vi "GUI RMM List.vi"(7 "FOFB-Controller IP Address in":string, 8 "error in (no error)":errorcluster, 9 "directory path":string, 10 "username":string, 11 "password":string) -> (0 "error out":errorcluster, 3 "RMM List":string[](array[string]))   [LabVIEW 2011, in "User Interface VIs.lvlib"]
uses:
  User Interface VIs.lvlib
  <vilib>/addons/internet/NI_InternetTK_FTP_VIs.lvlib
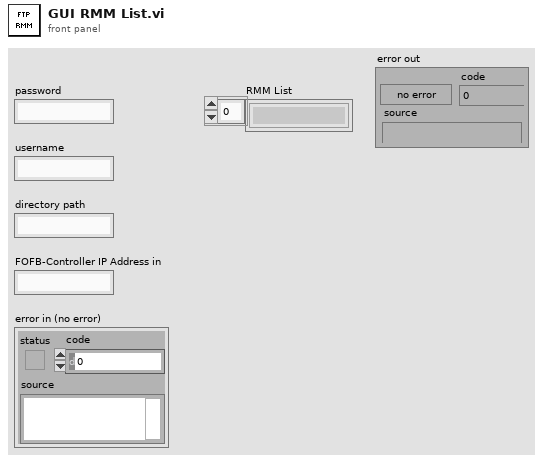
[diagram p1: front panel]
types:
  T1 = typedef "FTP Session.ctl" = refnum<k1>
  T2 = typedef "FTP File Info.ctl" = cluster{"type":enum16{"unknown", "file", "dir", "link"}, "permissions":string, "owner":string, "group":string, "size":i32, "date":string, "name":string, "link name":string}
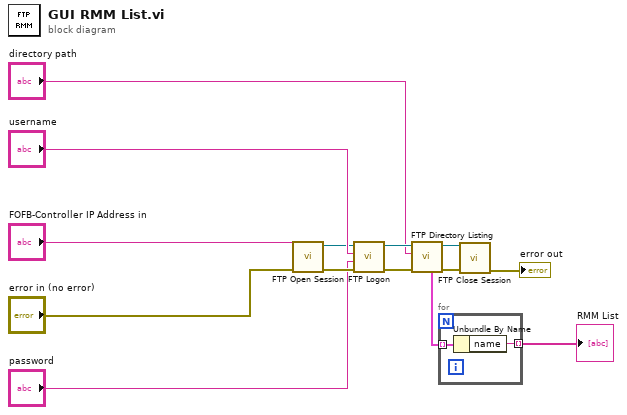
[diagram p0: block diagram]
diagram:
  n1 = call <vilib>:"FTP Open Session.vi"("error in (no error)"="error in (no error)", "address"="FOFB-Controller IP Address in") -> ("error out"=w12:errorcluster, "ftp session"=w5:T1)  [unwired: 6 in, 2 out]
  n2 = call <vilib>:"FTP Logon.vi"("error in (no error)"=w12, "password"="password", "user"="username", "ftp session"=w5) -> ("error out"=w13:errorcluster, "ftp session out"=w6:T1)  [unwired: 4 in, 2 out]
  n3 = call <vilib>:"FTP Directory Listing.vi"("error in (no error)"=w13, "directory path"="directory path", "ftp session"=w6) -> ("error out"=w14:errorcluster, "ftp session out"=w2:T1, "dir list"=w9:T2[])  [unwired: 4 in, 2 out]
  n4 = for {
    tunnel: w9 -> [w16] mode=indexing
    tunnel: [w15] -> w10 mode=indexing
    n5 = Unbundle By Name(w16) -> ("name"=w15:string)
  }
  "RMM List" <- w10
  n6 = call <vilib>:"FTP Close Session.vi"("error in (no error)"=w14, "ftp session"=w2) -> ("error out"=→"error out":errorcluster)  [unwired: 6 in, 3 out]
